vi "Oil.vi"(4 "Adjust":dbl, 6 "循环次数":i32, 7 "PreValue":dbl, 9 "ValueCal":bool, 10 "当前值":dbl, 11 "Seperation1.0":dbl) -> (3 "OilValue1":dbl format="%#.3f")   [LabVIEW 2014]
uses:
  <vilib>/ptbypt/NI_PtbyPt.lvlib
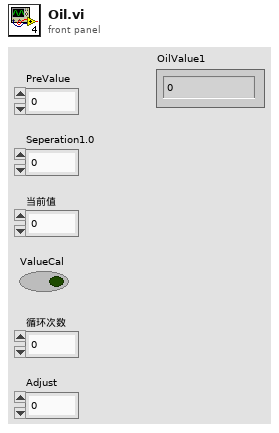
[diagram p1: front panel]
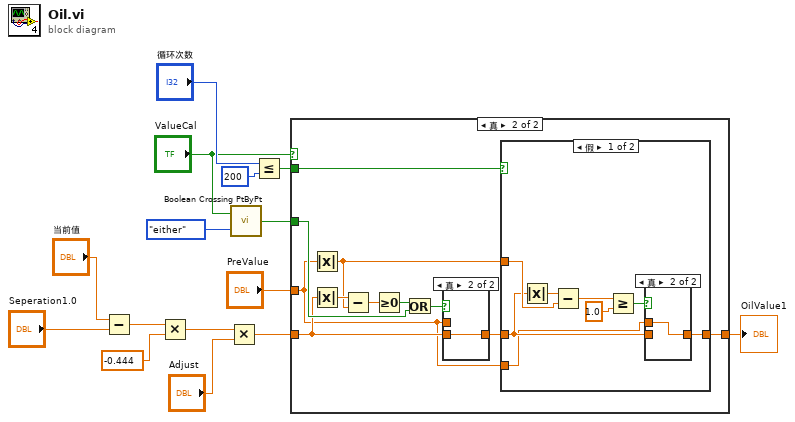
[diagram p0: block diagram]
diagram:
  n1 = Subtract(x="当前值", y="Seperation1.0") -> (x-y=w4:dbl)
  n2 = Multiply(x=w4, y=-0.444) -> (x*y=w8:dbl)
  n3 = Multiply(x=w8, y="Adjust") -> (x*y=w9:dbl)
  n4 = call <vilib>:"Boolean Crossing PtByPt.vi"("direction"=enum16{"either", "false-true", "true-false"}."either", "input"="ValueCal") -> ("crossing"=w7:bool)  [unwired: 1 in]
  n5 = Less Or Equal?(x="循环次数", y=200) -> (x <= y?=w2:bool)
  n6 = case shown="真" "ValueCal" {
    tunnel: w7 -> [_ w23]
    tunnel: w9 -> [w16 w22]
    tunnel: "PreValue" -> [_ w17]
    tunnel: [w16 w19] -> w11
    tunnel: w2 -> [_ w18]
    frame False {
    }
    frame True {
      n7 = Absolute Value(x=w17) -> (abs(x)=w21:dbl)
      n8 = Absolute Value(x=w22) -> (abs(x)=w27:dbl)
      n9 = Subtract(x=w27, y=w21) -> (x-y=w26:dbl)
      n10 = Greater Or Equal To 0?(x=w26) -> (x >= 0?=w25:bool)
      n11 = Or(x=w25, y=w23) -> (x .or. y?=w24:bool)
      n12 = case shown="真" w24 {
        tunnel: w22 -> [_ w40]
        tunnel: [w39 w40] -> w20
        tunnel: w17 -> [w39 _]
        frame False {
        }
        frame True {
        }
      }
      n13 = case shown="假" w18 {
        tunnel: w21 -> [w34 _]
        tunnel: w20 -> [w30 w38]
        tunnel: [w29 w38] -> w19
        tunnel: w17 -> [w28 _]
        frame False {
          n14 = Absolute Value(x=w30) -> (abs(x)=w35:dbl)
          n15 = Subtract(x=w35, y=w34) -> (x-y=w33:dbl)
          n16 = Greater Or Equal?(x=w33, y=1.0) -> (x >= y?=w31:bool)
          n17 = case shown="真" w31 {
            tunnel: w30 -> [w36 _]
            tunnel: [w36 w37] -> w29
            tunnel: w28 -> [_ w37]
            frame False {
            }
            frame True {
            }
          }
        }
        frame True {
        }
      }
    }
  }
  "OilValue1" <- w11
